vi "CountAndScan_v3.vi"() -> ()   [LabVIEW 2010]
uses:
  <vilib>/Utility/file.llb/Write To Spreadsheet File (DBL).vi
panel:
  out "Current-Calculated2":dbl caption="Current"
  out "Current-Calculated1":dbl caption="Current"
  in  "Timer":dbl=30.0 min=0.0 step=1.0
  out "Timer Progress":u8(slide)=29 scale=-1.1..4.0
  in  "SendMailAtEnd":bool=TRUE caption="at End"
  in  "SendMailAtEach":bool=TRUE caption="at Each Point"
  in  "SendMailAtStart":bool caption="at Start"
  out "Complete 2?":bool
  out "Homed ? 2":bool=TRUE caption="Homed ?"
  in  "MG17Motor 2":refnum<k7>(container)
  out "plStatusBits 2":i32=-1341913856
  out "Motor 2 error":errorcluster
  out "Motor 2":refnum<k7>
  out "plStatusBits":i32=-1341913856
  out "Homed ?":bool=TRUE
  out "Motor 1 error":errorcluster
  out "Motor 1":refnum<k7>
  in  "Beep":u16(ring)=1 items=["Off", "Each point", "End"]
  out "Aux":u64[](array[numeric])=[1279, 1631, 0]
  out "path":path=path "D:/Documents and Settings/All Users/Marcelo/Medidas/Paridade/2013-11-14 BBO/2013-11-13_97_placa_0.08gr_1200s.txt"
  out "Target 2":dbl caption="Target" format="%.2g"
  out "Current 2":sgl caption="APT-Current" format="%.2g"
  in  "Step 2":dbl caption="Step" min=0.3 max=360.0 step=1.0
  in  "Stop 2":dbl=50.0 caption="Stop" min=0.0 max=360.0 step=1.0
  in  "Start 2":dbl caption="Start" min=0.0 max=360.0 step=1.0
  out "Count 33":u32
  out "Count 32":u32
  out "Count 31":u32
  out "Count 23":u32
  out "Count 22":u32
  out "Count 21":u32
  out "Count 13":u32
  out "Count 12":u32=1631
  out "Count 11":u32=1279
  in  "stop":bool
  out "Target":dbl=19.0 format="%.2g"
  out "Complete 1?":bool=TRUE
  out "# of steps":dbl
  out "Current":sgl=18.999899 caption="APT-Current" format="%.2g"
  in  "Step":dbl=0.07999999821186066 min=0.02 max=360.0 step=1.0
  in  "Stop":dbl=19.08 min=0.0 max=360.0 step=1.0
  in  "Start":dbl=19.0 min=0.0 max=360.0 step=1.0
  in  "Serial Motor 2":i32=83829605 min=0 step=1
  in  "Serial Motor 1":i32=83830377 min=0 step=1
  in  "MG17Motor":refnum<k7>(container)
  out "ByteSize":u8=4
  in  "Sampling time":dbl=1200.0 min=0.0 step=1.0
  out "Handle 3":u32
  out "size(s)":i32=3
  out "Waveform Chart 9":u32(graph)
  out "Waveform Chart 8":u32(graph)
  out "Waveform Chart 7":u32(graph)
  out "Waveform Chart 6":u32(graph)
  out "Waveform Chart 5":u32(graph)
  out "Waveform Chart 4":u32(graph)
  out "Waveform Chart 3":u32(graph)
  out "Waveform Chart 2":u32(graph)=1631
  out "Waveform Chart 1":u32(graph)=1279
  in  "Plot 9":string(combo)="14"
  in  "Plot 8":string(combo)="8"
  in  "Plot 7":string(combo)="7"
  in  "Plot 6":string(combo)="6"
  in  "Plot 5":string(combo)="4"
  in  "Plot 4":string(combo)="3"
  in  "Plot 3":string(combo)="2"
  in  "Plot 2":string(combo)="1"
  in  "Plot 1":string(combo)="0"
  out "Delcom Serial Number":u32=20844 caption="20861"
  out "Handle":u32=17176
  out "2D Scan":bool
  out "Scan 2":bool
  out "Scan 1":bool=TRUE
  in  "Slide":dbl(slide)=1.0 min=0.0 max=2.0 step=1.0 scale=0.0..2.0
  in  "APD 4":bool
  in  "APD 3":bool
  in  "APD 2":bool=TRUE
  in  "APD 1":bool=TRUE
  # "FPGA SERIAL NUMBER"
  # "MOTOR 1"
  # "MOTOR 2"
  # "Send email"
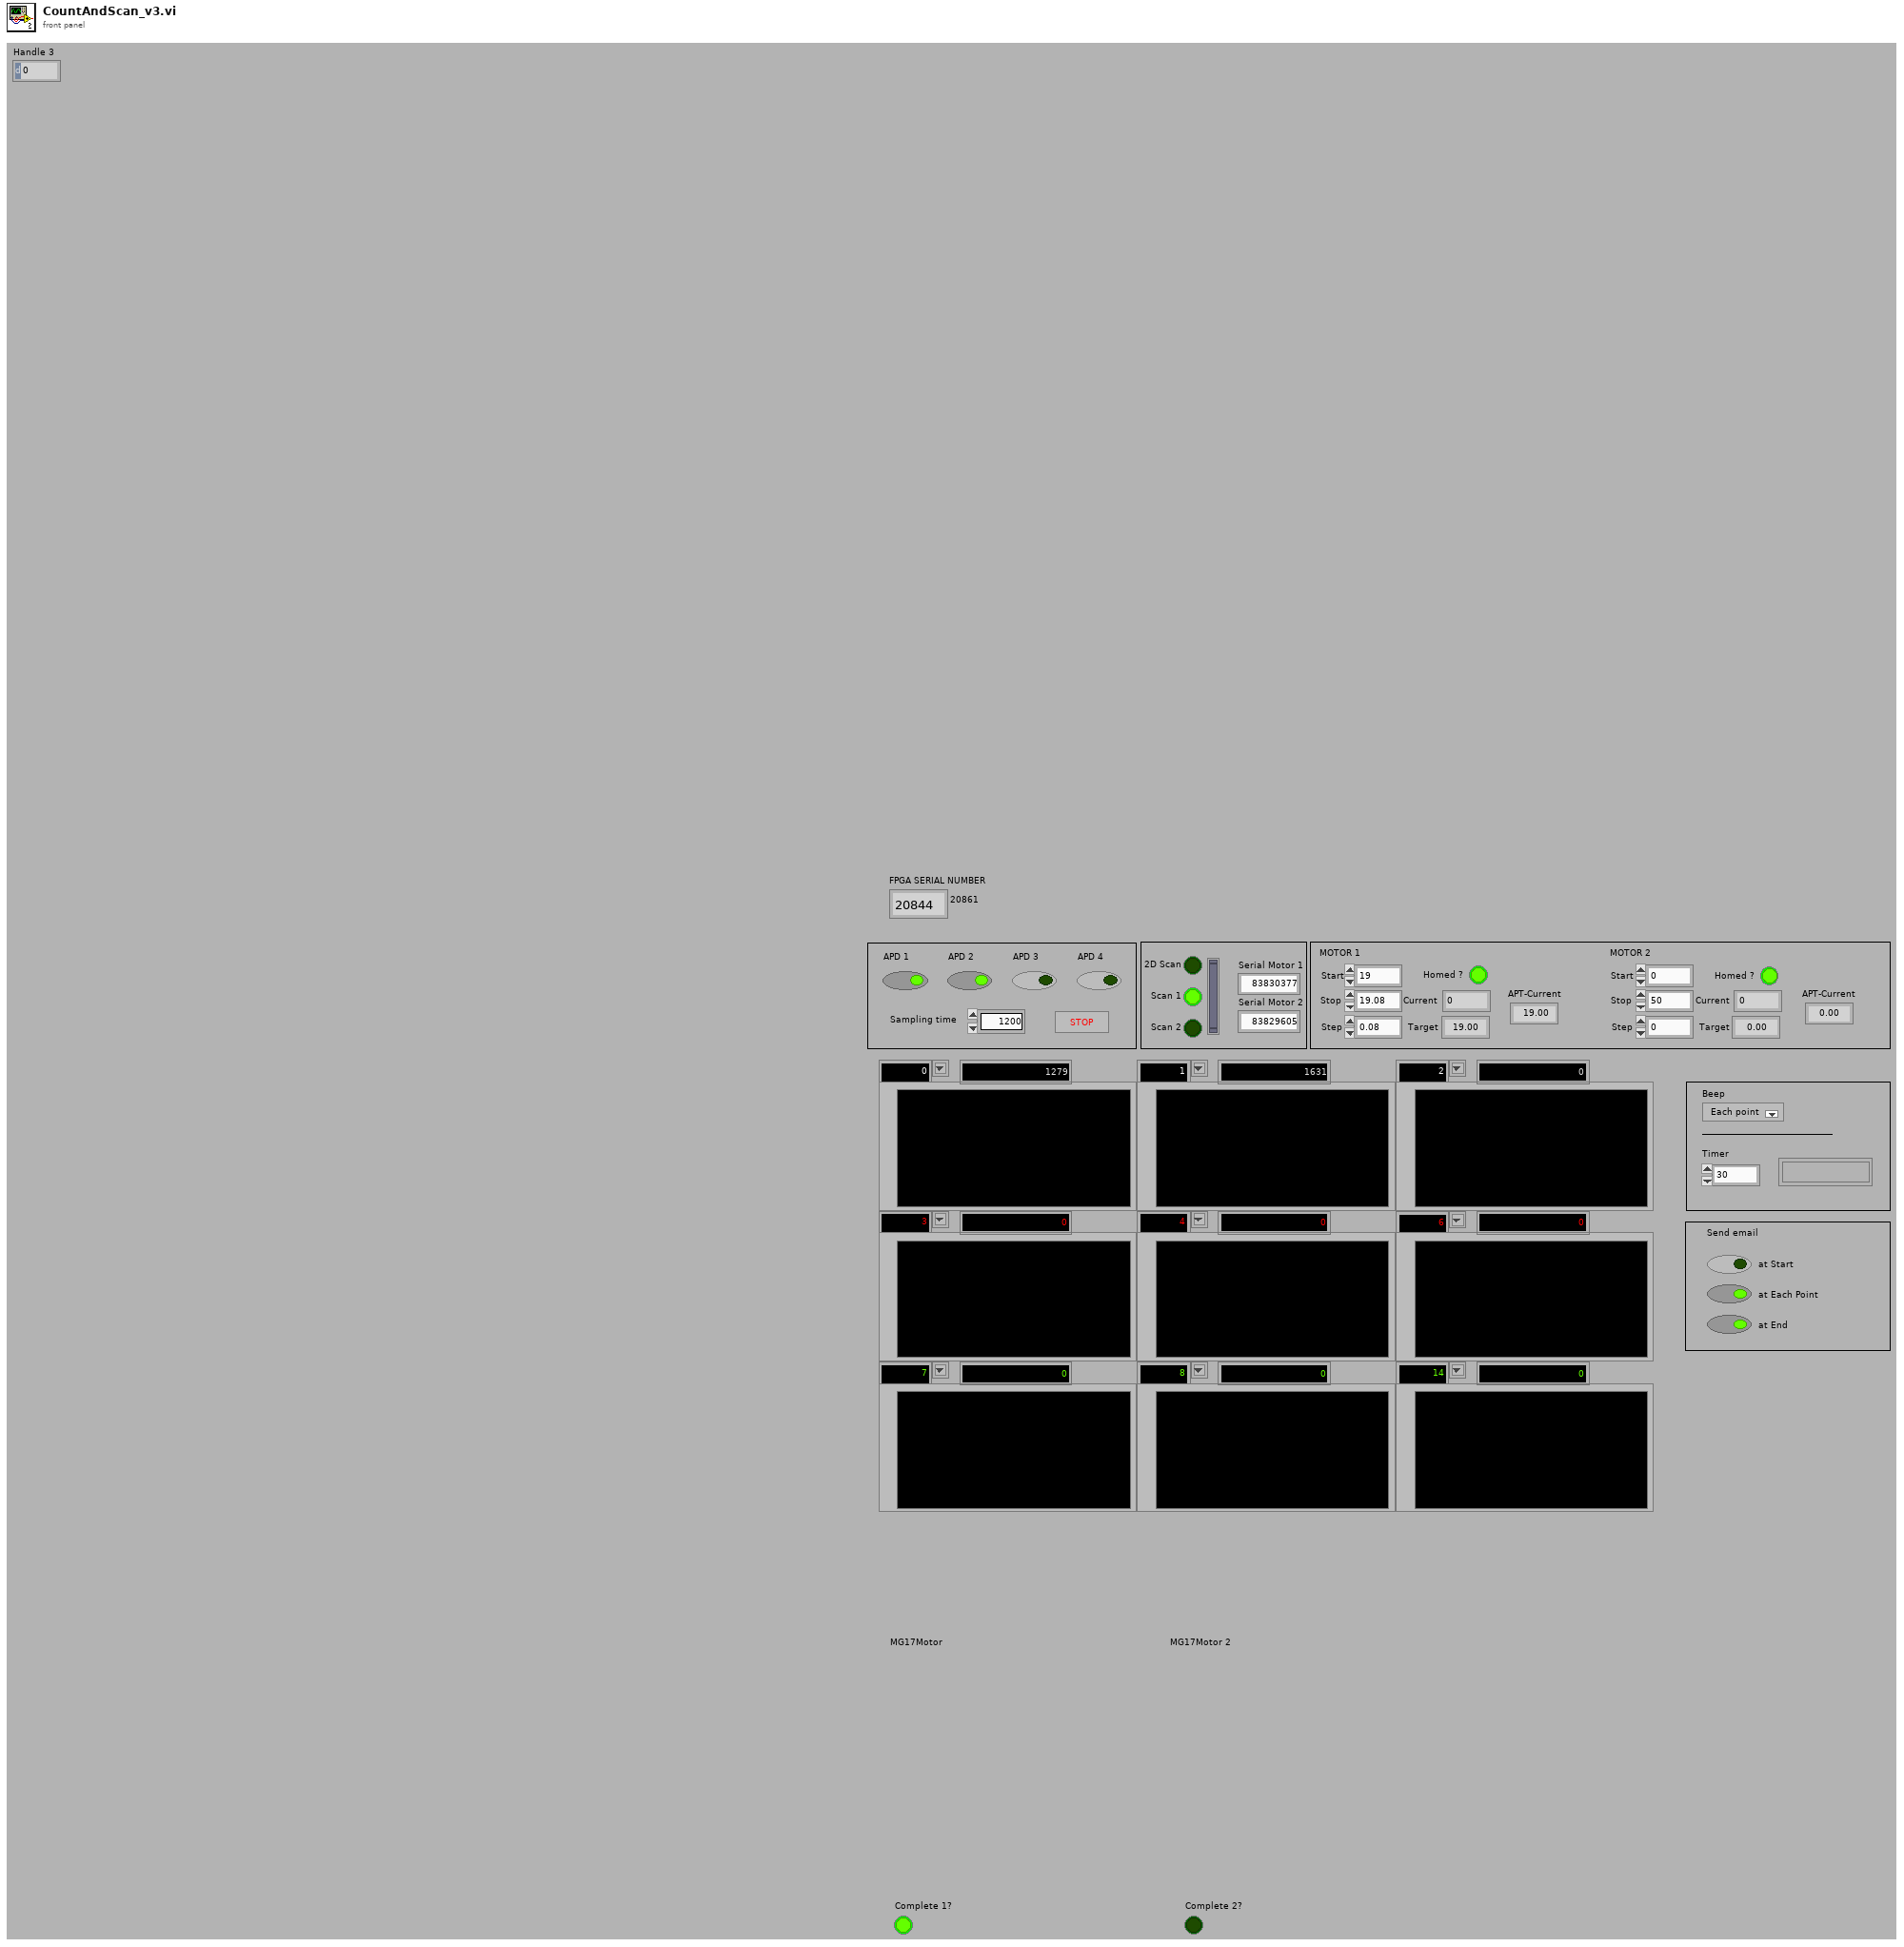
[diagram p1: front panel]
types:
  T1 = enum8{"Enabled", "Disabled", "Disabled and Grayed Out"}
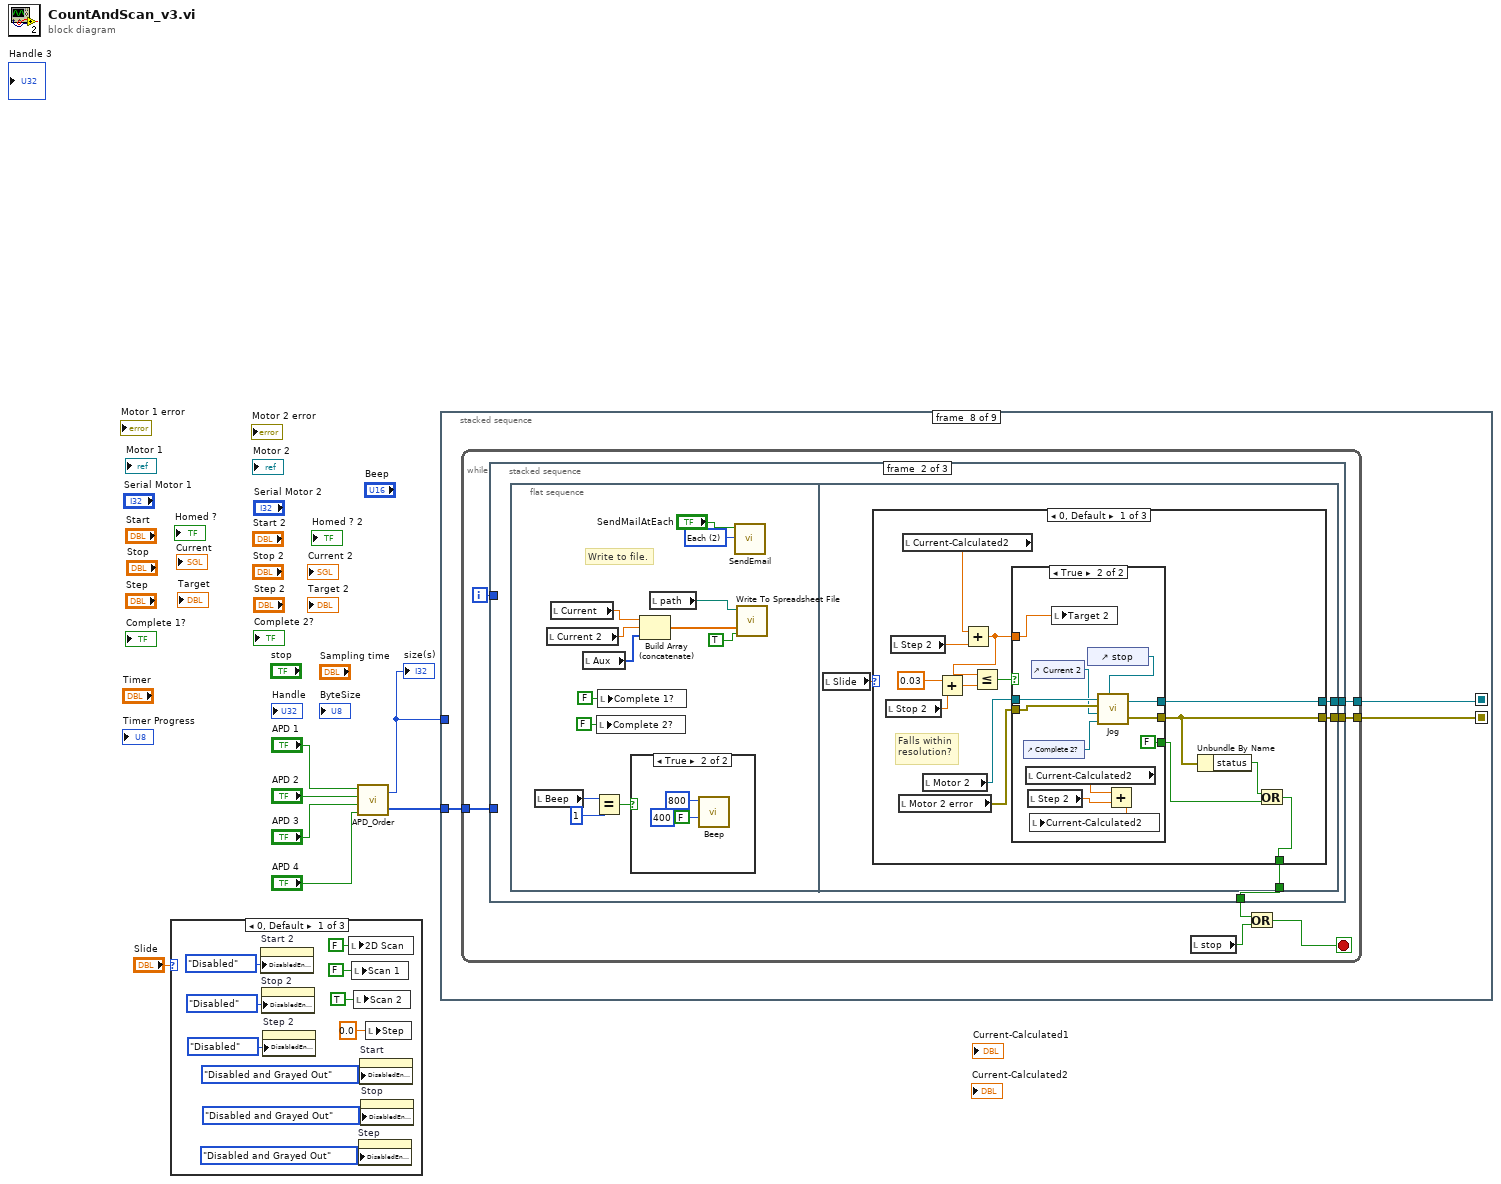
[diagram p0: block diagram]
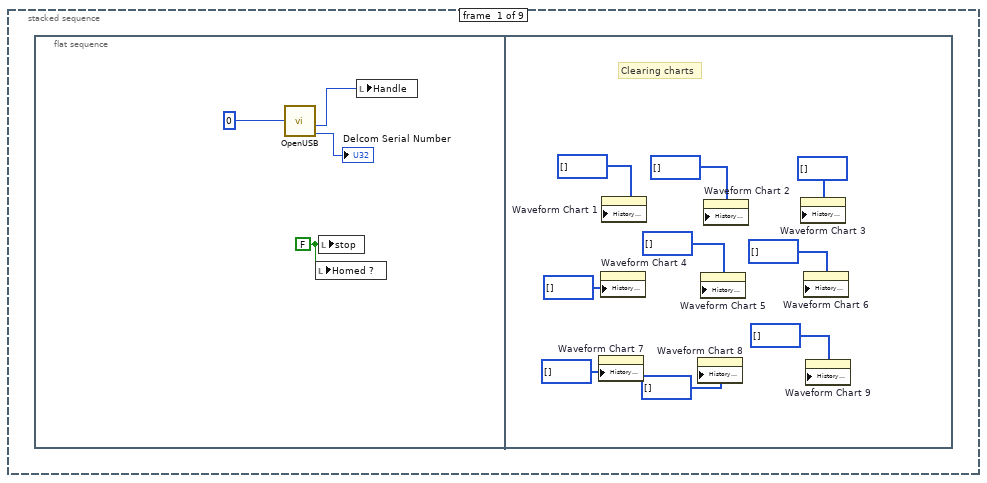
[diagram p2: hidden frame]
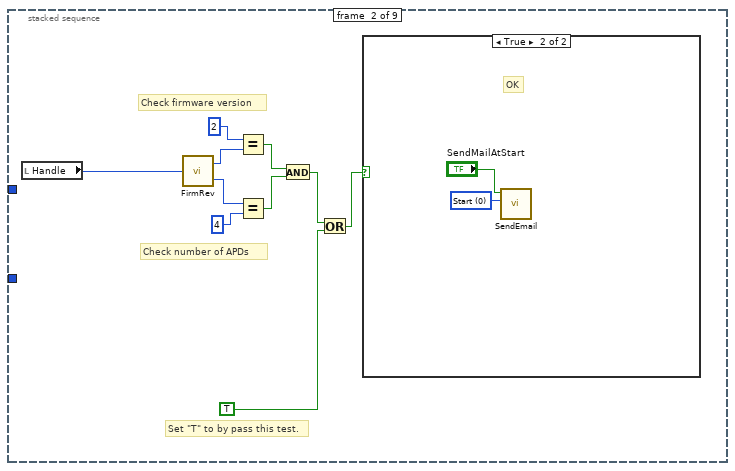
[diagram p3: hidden frame]
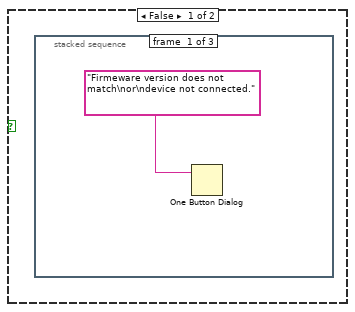
[diagram p4: hidden frame]
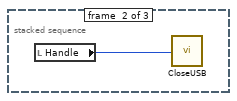
[diagram p5: hidden frame]
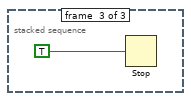
[diagram p6: hidden frame]
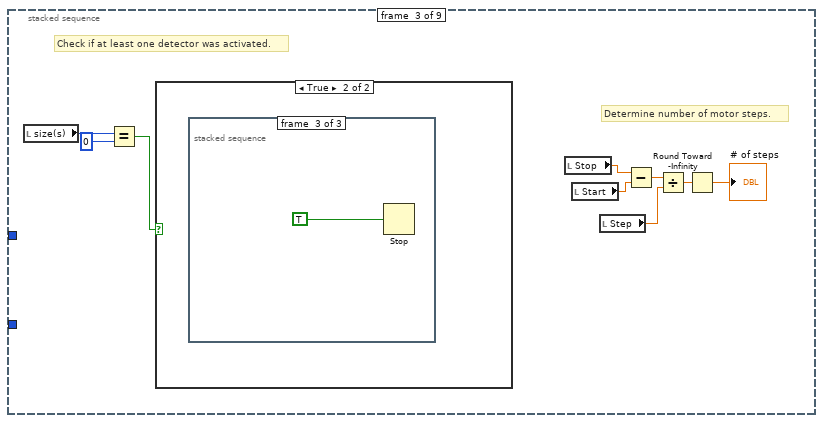
[diagram p7: hidden frame]
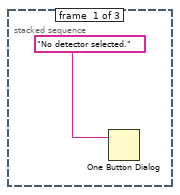
[diagram p9: hidden frame]
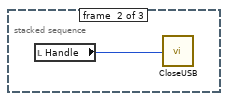
[diagram p10: hidden frame]
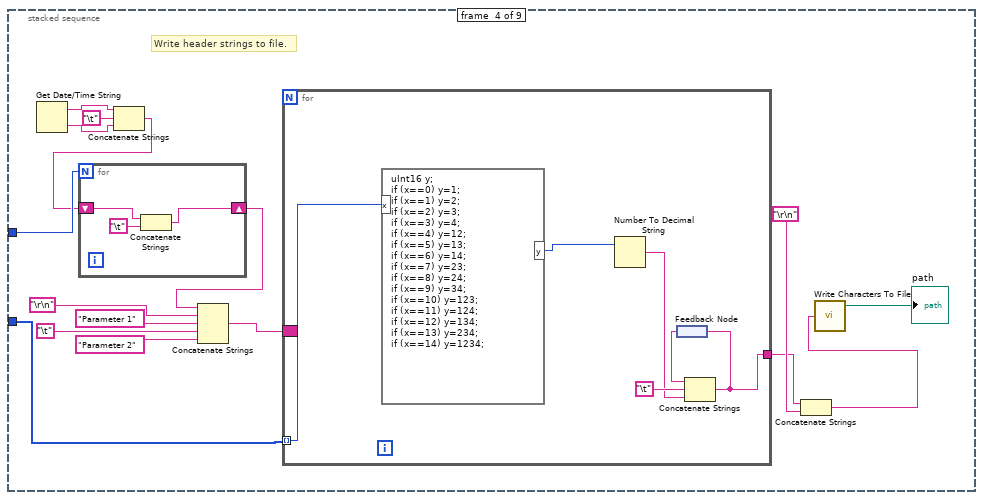
[diagram p11: hidden frame]
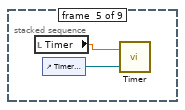
[diagram p12: hidden frame]
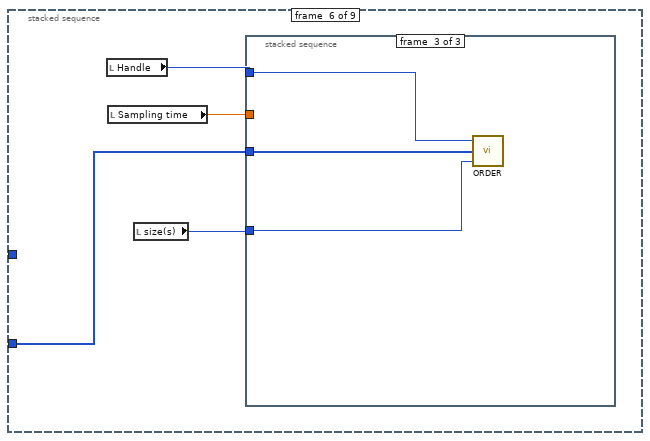
[diagram p13: hidden frame]
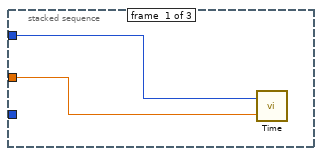
[diagram p14: hidden frame]
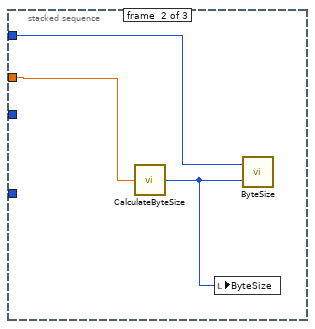
[diagram p15: hidden frame]
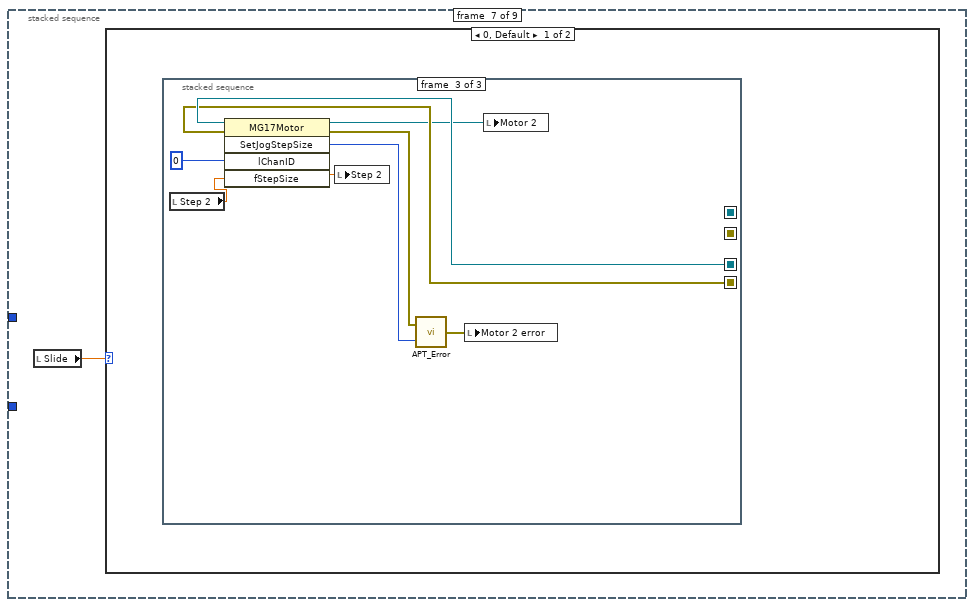
[diagram p16: hidden frame]
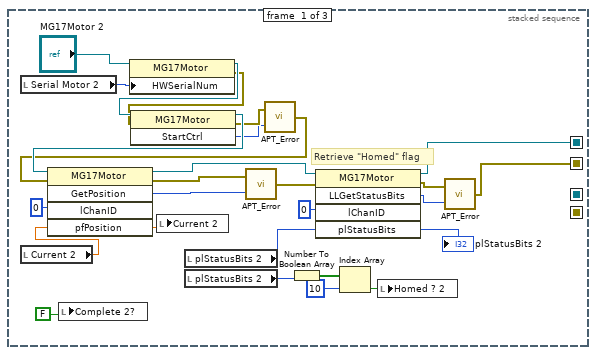
[diagram p17: hidden frame]
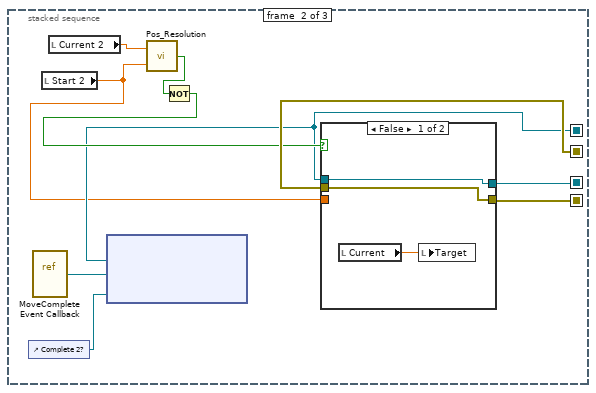
[diagram p18: hidden frame]
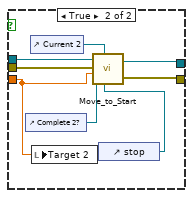
[diagram p19: hidden frame]
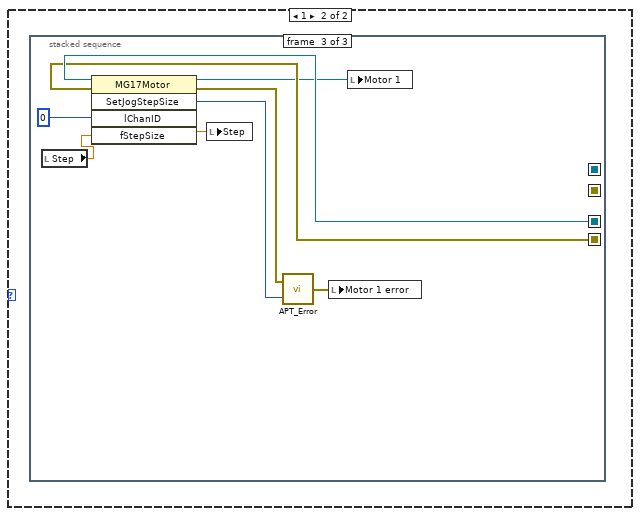
[diagram p20: hidden frame]
diagram:
  n1 = case shown="0, Default" "Slide" {
    frame 0, Default {
      n2 = property on="Start 2" class="DigNum (strict)"("DisabledEnum"=T1."Disabled" ("Disabled")) -> ()  [unwired: 2 in, 2 out]
      n3 = property on="Stop 2" class="DigNum (strict)"("DisabledEnum"=T1."Disabled" ("Disabled")) -> ()  [unwired: 2 in, 2 out]
      n4 = property on="Step 2" class="DigNum (strict)"("DisabledEnum"=T1."Disabled" ("Disabled")) -> ()  [unwired: 2 in, 2 out]
      n5 = local write "2D Scan"(FALSE ("Manual")) -> ()
      n6 = local write "Scan 1"(FALSE ("Scan 1")) -> ()
      n7 = local write "Scan 2"(TRUE ("Scan 2")) -> ()
      n8 = property on="Step" class="DigNum (strict)"("DisabledEnum"=T1."Disabled and Grayed Out" ("Disabled")) -> ()  [unwired: 2 in, 2 out]
      n9 = property on="Start" class="DigNum (strict)"("DisabledEnum"=T1."Disabled and Grayed Out" ("Disabled")) -> ()  [unwired: 2 in, 2 out]
      n10 = property on="Stop" class="DigNum (strict)"("DisabledEnum"=T1."Disabled and Grayed Out" ("Disabled")) -> ()  [unwired: 2 in, 2 out]
      n11 = local write "Step"(0.0 ("Step")) -> ()
    }
    frame 1 {
      n12 = property on="Start" class="DigNum (strict)"("DisabledEnum"=T1."Disabled" ("Disabled")) -> ()  [unwired: 2 in, 2 out]
      n13 = property on="Stop" class="DigNum (strict)"("DisabledEnum"=T1."Disabled" ("Disabled")) -> ()  [unwired: 2 in, 2 out]
      n14 = property on="Step" class="DigNum (strict)"("DisabledEnum"=T1."Disabled" ("Disabled")) -> ()  [unwired: 2 in, 2 out]
      n15 = property on="Start 2" class="DigNum (strict)"("DisabledEnum"=T1."Disabled and Grayed Out" ("Disabled")) -> ()  [unwired: 2 in, 2 out]
      n16 = property on="Stop 2" class="DigNum (strict)"("DisabledEnum"=T1."Disabled and Grayed Out" ("Disabled")) -> ()  [unwired: 2 in, 2 out]
      n17 = property on="Step 2" class="DigNum (strict)"("DisabledEnum"=T1."Disabled and Grayed Out" ("Disabled")) -> ()  [unwired: 2 in, 2 out]
      n18 = local write "Step 2"(0.0 ("Step 2")) -> ()
      n19 = local write "Scan 2"(FALSE ("Scan 2")) -> ()
      n20 = local write "2D Scan"(FALSE ("Manual")) -> ()
      n21 = local write "Scan 1"(TRUE ("Scan 1")) -> ()
    }
    frame 2 {
      "Scan 1" <- FALSE ("Scan 1")
      "2D Scan" <- TRUE ("Manual")
      "Scan 2" <- FALSE ("Scan 2")
    }
  }
  n22 = call "APD_Order.vi"("APD 4"="APD 4", "APD 3"="APD 3", "APD 2"="APD 2", "APD 1"="APD 1") -> ("Detectors"=w1:i32[], "size(s)"=w2:i32)
  "size(s)" <- w2
  n23 = stacked-sequence {
    seq-local: [_ _ _ _ _ _ _ w226 _] -> [_ _ _ _ _ _ _ _ w354]
    seq-local: [_ _ _ _ _ _ _ w225 _] -> [_ _ _ _ _ _ _ _ w353]
    tunnel: w2 -> [_ _ _ w80 _ _ _ _ _]
    tunnel: w1 -> [_ _ _ w73 _ w99 _ w227 _]
    frame #0 {
      n24 = flat-sequence {
        frame #0 {
          w31 = FALSE ("stop")
          n25 = call "OpenUSB.vi"("Device Number"=u32 0) -> ("Handle"=w32:u32, "Delcom Serial Number"=→"Delcom Serial Number":u32)  [unwired: 2 out]
          n26 = local write "Homed ?"(w31) -> ()
          n27 = local write "stop"(w31) -> ()
          n28 = local write "Handle"(w32) -> ()
        }
        frame #1 {
          # "Clearing charts"
          n29 = property on="Waveform Chart 7" class="WFChart (strict)"("History Data"=i32[] []) -> ()  [unwired: 2 in, 2 out]
          n30 = property on="Waveform Chart 4" class="WFChart (strict)"("History Data"=i32[] []) -> ()  [unwired: 2 in, 2 out]
          n31 = property on="Waveform Chart 1" class="WFChart (strict)"("History Data"=i32[] []) -> ()  [unwired: 2 in, 2 out]
          n32 = property on="Waveform Chart 8" class="WFChart (strict)"("History Data"=i32[] []) -> ()  [unwired: 2 in, 2 out]
          n33 = property on="Waveform Chart 5" class="WFChart (strict)"("History Data"=i32[] []) -> ()  [unwired: 2 in, 2 out]
          n34 = property on="Waveform Chart 2" class="WFChart (strict)"("History Data"=i32[] []) -> ()  [unwired: 2 in, 2 out]
          n35 = property on="Waveform Chart 3" class="WFChart (strict)"("History Data"=i32[] []) -> ()  [unwired: 2 in, 2 out]
          n36 = property on="Waveform Chart 6" class="WFChart (strict)"("History Data"=i32[] []) -> ()  [unwired: 2 in, 2 out]
          n37 = property on="Waveform Chart 9" class="WFChart (strict)"("History Data"=i32[] []) -> ()  [unwired: 2 in, 2 out]
        }
      }
    }
    frame #1 {
      # "Set \"T\" to by pass this test."
      # "Check number of APDs"
      # "Check firmware version"
      n38 = local read "Handle"() -> (w44:u32)
      n39 = call "FirmRev.vi"("Handle"=w44) -> ("Firmeware Version"=w45:u8, "APD nunmber"=w46:u8)
      n40 = Equal?(x=u8 2, y=w45) -> (x = y?=w49:bool)
      n41 = Equal?(x=w46, y=u8 4) -> (x = y?=w50:bool)
      n42 = And(x=w49, y=w50) -> (x .and. y?=w51:bool)
      n43 = Or(x=w51, y=TRUE) -> (x .or. y?=w52:bool)
      n44 = case shown="True" w52 {
        frame False {
          n45 = stacked-sequence {
            frame #0 {
              n46 = One Button Dialog(message="Firmeware version does not match\nor\ndevice not connected.") -> ()  [unwired: 1 in, 1 out]
            }
            frame #1 {
              n47 = local read "Handle"() -> (w55:u32)
              n48 = call "CloseUSB.vi"("Handle"=w55) -> ()  [unwired: 1 out]
            }
            frame #2 {
              n49 = Stop(stop? (T)=TRUE) -> ()
            }
          }
        }
        frame True {
          w58 = u16 0 items=["Start", "Stop", "Each"] ("Ring")
          # "OK"
          n50 = call "SendEmail.vi"("Send?"="SendMailAtStart", "Ring"=w58) -> ()  [unwired: 5 in]
        }
      }
    }
    frame #2 {
      # "Determine number of motor steps."
      # "Check if at least one detector was activated."
      n51 = local read "size(s)"() -> (w67:i32)
      n52 = Equal?(x=w67, y=0) -> (x = y?=w65:bool)
      n53 = case shown="True" w65 {
        frame False {
          # "PASS"
        }
        frame True {
          n54 = stacked-sequence {
            frame #0 {
              n55 = One Button Dialog(message="No detector selected.") -> ()  [unwired: 1 in, 1 out]
            }
            frame #1 {
              n56 = local read "Handle"() -> (w69:u32)
              n57 = call "CloseUSB.vi"("Handle"=w69) -> ()  [unwired: 1 out]
            }
            frame #2 {
              n58 = Stop(stop? (T)=TRUE) -> ()
            }
          }
        }
      }
      n59 = local read "Stop"() -> (w59:dbl)
      n60 = local read "Start"() -> (w64:dbl)
      n61 = local read "Step"() -> (w62:dbl)
      n62 = Subtract(x=w59, y=w64) -> (x-y=w63:dbl)
      n63 = Divide(x=w63, y=w62) -> (x/y=w61:dbl)
      n64 = Round Toward -Infinity(1:w61) -> (0:→"# of steps":dbl)
    }
    frame #3 {
      # "Write header strings to file."
      n65 = Get Date/Time String() -> (date string=w81:string, time string=w82:string)  [unwired: 3 in]
      n66 = Concatenate Strings(w81, "\t", w82) -> (w79:string)
      n67 = for {
        N: w80 -> [_]
        shift-right: [w94] -> w77
        shift-left: w79 -> [w93]
        n68 = Concatenate Strings(w93, "\t") -> (w94:string)
      }
      n69 = Concatenate Strings(w77, "\r\n", "Parameter 1", "\t", "Parameter 2") -> (w72:string)
      n70 = for {
        tunnel: [w91] -> w75
        border: w72 -> [_]
        tunnel: w73 -> [w87] mode=indexing
        n71 = formula code="uInt16 y;\nif (x==0) y=1;\nif (x==1) y=2;\nif (x==2) y=3;\nif (x==3) y=4;\nif (x==4) y=12;\nif (x==5) y=13;\nif (x==6) y=14;\nif (x==7) y=23;\nif (x==8) y=24;\nif (x==9) y=34;\nif (x==10) y=123;\nif (x==11) y=124;\nif (x==12) y=134;\nif (x==13) y=234;\nif (x==14) y=1234;"("x"=w87) -> ("y"=w89:u16)
        n72 = Number To Decimal String(number=w89) -> (decimal integer string=w88:string)  [unwired: 1 in]
        n73 = feedback #1() -> (w92:string)
        n74 = Concatenate Strings(w92, "\t", w88) -> (w91:string)
        n75 = feedback-in #1(w91) -> ()
      }
      n76 = Concatenate Strings(w75, "\r\n") -> (w74:string)
      n77 = call <vilib>:"Write Characters To File.vi"("character string"=w74) -> ("new file path (Not A Path if cancelled)"=→"path":path)  [unwired: 4 in]
    }
    frame #4 {
      n78 = local read "Timer"() -> (w96:dbl)
      n79 = control-ref of="Timer Progress"() -> (w97:refnum<vi>)
      n80 = call "Timer.vi"("Timer Progress"=w97, "Timer"=w96) -> ()  [unwired: 1 in]
    }
    frame #5 {
      n81 = local read "Handle"() -> (w101:u32)
      n82 = local read "Sampling time"() -> (w98:dbl)
      n83 = local read "size(s)"() -> (w100:i32)
      n84 = stacked-sequence {
        tunnel: w101 -> [w103 w106 w109]
        tunnel: w100 -> [_ _ w108]
        tunnel: w98 -> [w102 w105 _]
        tunnel: w99 -> [_ _ w107]
        frame #0 {
          n85 = call "Time.vi"("Time (s)"=w102, "Handle"=w103) -> ()  [unwired: 1 in]
        }
        frame #1 {
          n86 = call "CalculateByteSize.vi"("Tempo (s)"=w105) -> ("ByteSize"=w104:u8)
          n87 = local write "ByteSize"(w104) -> ()
          n88 = call "ByteSize.vi"("CounterByteSize"=w104, "Handle"=w106) -> ()  [unwired: 1 in]
        }
        frame #2 {
          n89 = call "ORDER.vi"("N"=w108, "Counter order"=w107, "Handle"=w109) -> ()  [unwired: 1 in]
        }
      }
    }
    frame #6 {
      n90 = local read "Slide"() -> (w110:dbl)
      n91 = case shown="0, Default" w110 {
        frame 0, Default {
          n92 = stacked-sequence {
            seq-local: [w119 _ _] -> [_ w141 _]
            seq-local: [w118 _ _] -> [_ w146 _]
            seq-local: [_ w143 _] -> [_ _ w167]
            seq-local: [_ w142 _] -> [_ _ w166]
            frame #0 {
              # "Retrieve \"Homed\" flag"
              n93 = local read "Serial Motor 2"() -> (w125:i32)
              n94 = local read "Current 2"() -> (w132:sgl)
              n95 = local write "Complete 2?"(FALSE ("Complete 1?")) -> ()
              n96 = property class="MG17Motor"(reference="MG17Motor 2", "HWSerialNum"=w125) -> (reference out=w136:refnum<k7>, error out=w135:errorcluster)  [unwired: 1 in]
              n97 = invoke class="MG17Motor" method="StartCtrl"(reference=w136, error in=w135) -> (reference out=w134:refnum<k7>, error out=w131:errorcluster, "StartCtrl"=w130:i32)  [unwired: 1 in]
              n98 = local read "plStatusBits 2"() -> (w113:i32)
              n99 = local read "plStatusBits 2"() -> (w111:i32)
              n100 = call "APT_Error.vi"("Return Code"=w130, "error in (no error)"=w131) -> ("error out"=w129:errorcluster)
              n101 = invoke class="MG17Motor" method="GetPosition"(reference=w134, error in=w129, "lChanID"=0, "pfPosition"=w132) -> (reference out=w123:refnum<k7>, error out=w128:errorcluster, "GetPosition"=w127:i32, "pfPosition"=w126:sgl)  [unwired: 1 in, 1 out]
              n102 = local write "Current 2"(w126) -> ()
              n103 = call "APT_Error.vi"("Return Code"=w127, "error in (no error)"=w128) -> ("error out"=w122:errorcluster)
              n104 = Number To Boolean Array(number=w111) -> (Boolean array=w116:bool[])
              n105 = invoke class="MG17Motor" method="LLGetStatusBits"(reference=w123, error in=w122, "lChanID"=0, "plStatusBits"=w113) -> (reference out=w119:refnum<k7>, error out=w120:errorcluster, "LLGetStatusBits"=w121:i32, "plStatusBits"=→"plStatusBits 2":i32)  [unwired: 1 in, 1 out]
              n106 = Index Array(array=w116, index=10) -> (element=w112:bool)
              n107 = local write "Homed ? 2"(w112) -> ()
              n108 = call "APT_Error.vi"("Return Code"=w121, "error in (no error)"=w120) -> ("error out"=w118:errorcluster)
            }
            frame #1 {
              n109 = control-ref of="Complete 2?"() -> (w140:refnum<vi>)
              n110 = vi-ref "MoveComplete Event Callback.vi"() -> ("vi reference"=w139:refnum<vi>)
              n111 = local read "Start 2"() -> (w138:dbl)
              n112 = local read "Current 2"() -> (w147:sgl)
              n113 = node(w141, w139, w140) -> ()  [unwired: 2 in, 2 out]
              n114 = call "Pos_Resolution.vi"("Target"=w138, "Current"=w147) -> ("Within resolution?"=w145:bool)
              n115 = Not(x=w145) -> (.not. x?=w144:bool)
              n116 = case shown="False" w144 {
                tunnel: w141 -> [w150 w157]
                tunnel: w146 -> [w149 w158]
                tunnel: [w150 w155] -> w143
                tunnel: [w149 w154] -> w142
                tunnel: w138 -> [_ w152]
                frame False {
                  n117 = local read "Current"() -> (w148:sgl)
                  n118 = local write "Target"(w148) -> ()
                }
                frame True {
                  n119 = control-ref of="Complete 2?"() -> (w153:refnum<vi>)
                  n120 = control-ref of="Current 2"() -> (w156:refnum<vi>)
                  n121 = local write "Target 2"(w152) -> ()
                  n122 = control-ref of="stop"() -> (w151:refnum<vi>)
                  n123 = call "Move_to_Start.vi"("Stop"=w151, "Current Pos"=w156, "Complete?"=w153, "Move To"=w152, "error in (no error)"=w158, "MG17Motor"=w157) -> ("error out"=w154:errorcluster, "reference out"=w155:refnum<k7>)
                }
              }
            }
            frame #2 {
              n124 = local read "Step 2"() -> (w163:dbl)
              n125 = invoke class="MG17Motor" method="SetJogStepSize"(reference=w167, error in=w166, "lChanID"=0, "fStepSize"=w163) -> (reference out=w162:refnum<k7>, error out=w161:errorcluster, "SetJogStepSize"=w160:i32, "fStepSize"=w164:sgl)  [unwired: 1 in, 1 out]
              n126 = local write "Step 2"(w164) -> ()
              n127 = call "APT_Error.vi"("Return Code"=w160, "error in (no error)"=w161) -> ("error out"=w159:errorcluster)
              n128 = local write "Motor 2 error"(w159) -> ()
              n129 = local write "Motor 2"(w162) -> ()
            }
          }
        }
        frame 1 {
          n130 = stacked-sequence {
            seq-local: [w176 _ _] -> [_ w198 _]
            seq-local: [w175 _ _] -> [_ w203 _]
            seq-local: [_ w200 _] -> [_ _ w224]
            seq-local: [_ w199 _] -> [_ _ w223]
            frame #0 {
              # "Retrieve \"Homed\" flag"
              n131 = local read "Serial Motor 1"() -> (w182:i32)
              n132 = local read "Current"() -> (w189:sgl)
              n133 = local write "Complete 1?"(FALSE ("Complete 1?")) -> ()
              n134 = property class="MG17Motor"(reference="MG17Motor", "HWSerialNum"=w182) -> (reference out=w193:refnum<k7>, error out=w192:errorcluster)  [unwired: 1 in]
              n135 = invoke class="MG17Motor" method="StartCtrl"(reference=w193, error in=w192) -> (reference out=w191:refnum<k7>, error out=w188:errorcluster, "StartCtrl"=w187:i32)  [unwired: 1 in]
              n136 = local read "plStatusBits"() -> (w170:i32)
              n137 = local read "plStatusBits"() -> (w168:i32)
              n138 = call "APT_Error.vi"("Return Code"=w187, "error in (no error)"=w188) -> ("error out"=w186:errorcluster)
              n139 = invoke class="MG17Motor" method="GetPosition"(reference=w191, error in=w186, "lChanID"=0, "pfPosition"=w189) -> (reference out=w180:refnum<k7>, error out=w185:errorcluster, "GetPosition"=w184:i32, "pfPosition"=w183:sgl)  [unwired: 1 in, 1 out]
              n140 = local write "Current"(w183) -> ()
              n141 = call "APT_Error.vi"("Return Code"=w184, "error in (no error)"=w185) -> ("error out"=w179:errorcluster)
              n142 = Number To Boolean Array(number=w168) -> (Boolean array=w173:bool[])
              n143 = invoke class="MG17Motor" method="LLGetStatusBits"(reference=w180, error in=w179, "lChanID"=0, "plStatusBits"=w170) -> (reference out=w176:refnum<k7>, error out=w177:errorcluster, "LLGetStatusBits"=w178:i32, "plStatusBits"=→"plStatusBits":i32)  [unwired: 1 in, 1 out]
              n144 = Index Array(array=w173, index=10) -> (element=w169:bool)
              n145 = local write "Homed ?"(w169) -> ()
              n146 = call "APT_Error.vi"("Return Code"=w178, "error in (no error)"=w177) -> ("error out"=w175:errorcluster)
            }
            frame #1 {
              n147 = control-ref of="Complete 1?"() -> (w197:refnum<vi>)
              n148 = vi-ref "MoveComplete Event Callback.vi"() -> ("vi reference"=w196:refnum<vi>)
              n149 = local read "Start"() -> (w195:dbl)
              n150 = local read "Current"() -> (w204:sgl)
              n151 = node(w198, w196, w197) -> ()  [unwired: 2 in, 2 out]
              n152 = call "Pos_Resolution.vi"("Target"=w195, "Current"=w204) -> ("Within resolution?"=w202:bool)
              n153 = Not(x=w202) -> (.not. x?=w201:bool)
              n154 = case shown="True" w201 {
                tunnel: w198 -> [w207 w214]
                tunnel: w203 -> [w206 w215]
                tunnel: [w207 w212] -> w200
                tunnel: [w206 w211] -> w199
                tunnel: w195 -> [_ w209]
                frame False {
                  n155 = local read "Current"() -> (w205:sgl)
                  n156 = local write "Target"(w205) -> ()
                }
                frame True {
                  n157 = control-ref of="Complete 1?"() -> (w210:refnum<vi>)
                  n158 = control-ref of="Current"() -> (w213:refnum<vi>)
                  n159 = local write "Target"(w209) -> ()
                  n160 = control-ref of="stop"() -> (w208:refnum<vi>)
                  n161 = call "Move_to_Start.vi"("Stop"=w208, "Current Pos"=w213, "Complete?"=w210, "Move To"=w209, "error in (no error)"=w215, "MG17Motor"=w214) -> ("error out"=w211:errorcluster, "reference out"=w212:refnum<k7>)
                }
              }
            }
            frame #2 {
              n162 = local read "Step"() -> (w220:dbl)
              n163 = invoke class="MG17Motor" method="SetJogStepSize"(reference=w224, error in=w223, "lChanID"=0, "fStepSize"=w220) -> (reference out=w219:refnum<k7>, error out=w218:errorcluster, "SetJogStepSize"=w217:i32, "fStepSize"=w221:sgl)  [unwired: 1 in, 1 out]
              n164 = local write "Step"(w221) -> ()
              n165 = call "APT_Error.vi"("Return Code"=w217, "error in (no error)"=w218) -> ("error out"=w216:errorcluster)
              n166 = local write "Motor 1 error"(w216) -> ()
              n167 = local write "Motor 1"(w219) -> ()
            }
          }
        }
      }
    }
    frame #7 {
      n168 = while {
        tunnel: w227 -> [w233]
        tunnel: [w229] -> w226
        tunnel: [w228] -> w225
        i -> [w234]
        stop <- w230 stop-if-true
        n169 = stacked-sequence {
          tunnel: w234 -> [w255 _ _]
          tunnel: w233 -> [w245 _ _]
          tunnel: [_ w262 _] -> w232
          tunnel: [_ w261 _] -> w229
          tunnel: [_ w260 _] -> w228
          frame #0 {
            # "Updates photon counts indicators."
            n170 = local read "Sampling time"() -> (w258:dbl)
            n171 = local read "ByteSize"() -> (w257:u8)
            n172 = local read "size(s)"() -> (w256:i32)
            n173 = local read "Handle"() -> (w259:u32)
            n174 = call "COUNTandREAD.vi"("i"=w255, "Byte size"=w257, "Num. of Counters"=w256, "tempo (s)"=w258, "handle"=w259) -> ("Output"=w235:u64[])  [unwired: 1 in]
            "Aux" <- w235
            n175 = call "Get_Element.vi"("Search for string"="Plot 7", "Det. list"=w245, "Meas. Data"=w235) -> ("Output"=→"Waveform Chart 7" →"Count 31":u32)
            n176 = call "Get_Element.vi"("Search for string"="Plot 4", "Det. list"=w245, "Meas. Data"=w235) -> ("Output"=→"Waveform Chart 4" →"Count 21":u32)
            n177 = call "Get_Element.vi"("Search for string"="Plot 1", "Det. list"=w245, "Meas. Data"=w235) -> ("Output"=→"Waveform Chart 1" →"Count 11":u32)
            n178 = call "Get_Element.vi"("Search for string"="Plot 8", "Det. list"=w245, "Meas. Data"=w235) -> ("Output"=→"Waveform Chart 8" →"Count 32":u32)
            n179 = call "Get_Element.vi"("Search for string"="Plot 2", "Det. list"=w245, "Meas. Data"=w235) -> ("Output"=→"Waveform Chart 2" →"Count 12":u32)
            n180 = call "Get_Element.vi"("Search for string"="Plot 5", "Det. list"=w245, "Meas. Data"=w235) -> ("Output"=→"Waveform Chart 5" →"Count 22":u32)
            n181 = call "Get_Element.vi"("Search for string"="Plot 9", "Det. list"=w245, "Meas. Data"=w235) -> ("Output"=→"Waveform Chart 9" →"Count 33":u32)
            n182 = call "Get_Element.vi"("Search for string"="Plot 6", "Det. list"=w245, "Meas. Data"=w235) -> ("Output"=→"Waveform Chart 6" →"Count 23":u32)
            n183 = call "Get_Element.vi"("Search for string"="Plot 3", "Det. list"=w245, "Meas. Data"=w235) -> ("Output"=→"Waveform Chart 3" →"Count 13":u32)
          }
          frame #1 {
            n184 = flat-sequence {
              tunnel: [w281] -> w262
              tunnel: [w280] -> w261
              tunnel: [w279] -> w260
              frame #0 {
                w263 = u16 2 items=["Start", "Stop", "Each"] ("Ring")
                # "Write to file."
                n185 = local read "Beep"() -> (w268:u16)
                n186 = local read "Current 2"() -> (w272:sgl)
                n187 = local read "Current"() -> (w273:sgl)
                n188 = local read "Aux"() -> (w271:u64[])
                n189 = Equal?(x=w268, y=u16 1) -> (x = y?=w266:bool)
                n190 = local write "Complete 2?"(FALSE ("Complete 1?")) -> ()
                n191 = local write "Complete 1?"(FALSE ("Complete 1?")) -> ()
                n192 = case shown="True" w266 {
                  frame False {
                  }
                  frame True {
                    n193 = call <vilib>:"Beep.vi"("use system alert? (T)"=FALSE, "duration (msec)"=u32 400, "frequency (Hz)"=u32 800) -> ()  [unwired: 9 in]
                  }
                }
                n194 = Build Array (concatenate)(w273, w272, w271) -> (w270:sgl[])
                n195 = local read "path"() -> (w275:path)
                n196 = call "SendEmail.vi"("Send?"="SendMailAtEach", "Ring"=w263) -> ()  [unwired: 5 in]
                n197 = call-poly <vilib>:"Write To Spreadsheet File.vi"("append to file? (new file:F)"=TRUE, "1D data"=w270, "file path (dialog if empty)"=w275) -> ()  [unwired: 5 in, 1 out]
              }
              frame #1 {
                n198 = local read "Slide"() -> (w282:dbl)
                n199 = case shown="0, Default" w282 {
                  tunnel: [w287 w316 FALSE ("status")] -> w281
                  tunnel: [w291 w320 refnum<k7> refnum ("reference out")] -> w280
                  tunnel: [w290 w319 errorcluster {"status"=FALSE, "code"=0, "source"=""} ("error out")] -> w279
                  frame 0, Default {
                    # "Falls within\nresolution?"
                    n200 = local read "Stop 2"() -> (w285:dbl)
                    n201 = local read "Step 2"() -> (w296:dbl)
                    n202 = local read "Motor 2 error"() -> (w292:errorcluster)
                    n203 = local read "Current-Calculated2"() -> (w283:dbl)
                    n204 = local read "Motor 2"() -> (w293:refnum<k7>)
                    n205 = Add(x=0.03, y=w285) -> (x+y=w284:dbl)
                    n206 = Add(x=w283, y=w296) -> (x+y=w294:dbl)
                    n207 = Less Or Equal?(x=w294, y=w284) -> (x <= y?=w295:bool)
                    n208 = case shown="True" w295 {
                      tunnel: w294 -> [_ w303]
                      tunnel: w293 -> [w298 w311]
                      tunnel: w292 -> [w297 w310]
                      tunnel: [w298 w306] -> w291
                      tunnel: [w297 w305] -> w290
                      tunnel: [TRUE FALSE] -> w289
                      frame False {
                      }
                      frame True {
                        n209 = control-ref of="Complete 2?"() -> (w308:refnum<vi>)
                        n210 = local read "Current-Calculated2"() -> (w302:dbl)
                        n211 = local read "Step 2"() -> (w301:dbl)
                        n212 = control-ref of="Current 2"() -> (w309:refnum<vi>)
                        n213 = local write "Target 2"(w303) -> ()
                        n214 = control-ref of="stop"() -> (w307:refnum<vi>)
                        n215 = call "Jog.vi"("MG17Motor"=w311, "error in (no error)"=w310, "Current Pos"=w309, "Complete?"=w308, "Stop"=w307) -> ("reference out"=w306:refnum<k7>, "error out"=w305:errorcluster)
                        n216 = Add(x=w302, y=w301) -> (x+y=w300:dbl)
                        n217 = local write "Current-Calculated2"(w300) -> ()
                      }
                    }
                    n218 = Unbundle By Name(w290) -> ("status"=w288:bool)
                    n219 = Or(x=w288, y=w289) -> (x .or. y?=w287:bool)
                  }
                  frame 1 {
                    # "Falls within\nresolution?"
                    n220 = local read "Current-Calculated1"() -> (w312:dbl)
                    n221 = local read "Stop"() -> (w314:dbl)
                    n222 = local read "Step"() -> (w325:dbl)
                    n223 = local read "Motor 1 error"() -> (w321:errorcluster)
                    n224 = local read "Motor 1"() -> (w322:refnum<k7>)
                    n225 = Add(x=0.03, y=w314) -> (x+y=w313:dbl)
                    n226 = Add(x=w312, y=w325) -> (x+y=w323:dbl)
                    n227 = Less Or Equal?(x=w323, y=w313) -> (x <= y?=w324:bool)
                    n228 = case shown="True" w324 {
                      tunnel: w323 -> [_ w332]
                      tunnel: w322 -> [w327 w340]
                      tunnel: w321 -> [w326 w339]
                      tunnel: [w327 w335] -> w320
                      tunnel: [w326 w334] -> w319
                      tunnel: [TRUE FALSE] -> w318
                      frame False {
                      }
                      frame True {
                        n229 = local read "Current-Calculated1"() -> (w331:dbl)
                        n230 = control-ref of="Complete 1?"() -> (w337:refnum<vi>)
                        n231 = local read "Step"() -> (w330:dbl)
                        n232 = control-ref of="Current"() -> (w338:refnum<vi>)
                        n233 = local write "Target"(w332) -> ()
                        n234 = control-ref of="stop"() -> (w336:refnum<vi>)
                        n235 = call "Jog.vi"("MG17Motor"=w340, "error in (no error)"=w339, "Current Pos"=w338, "Complete?"=w337, "Stop"=w336) -> ("reference out"=w335:refnum<k7>, "error out"=w334:errorcluster)
                        n236 = Add(x=w331, y=w330) -> (x+y=w329:dbl)
                        n237 = local write "Current-Calculated1"(w329) -> ()
                      }
                    }
                    n238 = Unbundle By Name(w319) -> ("status"=w317:bool)
                    n239 = Or(x=w317, y=w318) -> (x .or. y?=w316:bool)
                  }
                  frame 2 {
                    # "Temporary code. It is to be modified when\nraster scan is included."
                  }
                }
              }
            }
          }
          frame #2 {
            n240 = Wait (ms)(milliseconds to wait=u32 1000) -> ()  [unwired: 1 out]
          }
        }
        n241 = local read "stop"() -> (w231:bool)
        n242 = Or(x=w232, y=w231) -> (x .or. y?=w230:bool)
      }
    }
    frame #8 {
      w345 = u16 1 items=["Start", "Stop", "Each"] ("Ring")
      n243 = local read "Beep"() -> (w352:u16)
      n244 = local read "stop"() -> (w348:bool)
      n245 = Not(x=w348) -> (.not. x?=w347:bool)
      n246 = Equal?(x=w352, y=u16 2) -> (x = y?=w350:bool)
      n247 = property on="Start" class="DigNum (strict)"("DisabledEnum"=T1."Enabled" ("Disabled")) -> ()  [unwired: 2 in, 2 out]
      n248 = property on="Stop" class="DigNum (strict)"("DisabledEnum"=T1."Enabled" ("Disabled")) -> ()  [unwired: 2 in, 2 out]
      n249 = property on="Step" class="DigNum (strict)"("DisabledEnum"=T1."Enabled" ("Disabled")) -> ()  [unwired: 2 in, 2 out]
      n250 = And(x=w350, y=w347) -> (x .and. y?=w349:bool)
      n251 = case shown="True" w349 {
        frame False {
        }
        frame True {
          n252 = call <vilib>:"Beep.vi"("use system alert? (T)"=FALSE, "duration (msec)"=u32 400, "frequency (Hz)"=u32 800) -> ()  [unwired: 9 in]
        }
      }
      n253 = local read "Handle"() -> (w361:u32)
      n254 = property on="Start 2" class="DigNum (strict)"("DisabledEnum"=T1."Enabled" ("Disabled")) -> ()  [unwired: 2 in, 2 out]
      n255 = property on="Step 2" class="DigNum (strict)"("DisabledEnum"=T1."Enabled" ("Disabled")) -> ()  [unwired: 2 in, 2 out]
      n256 = property on="Stop 2" class="DigNum (strict)"("DisabledEnum"=T1."Enabled" ("Disabled")) -> ()  [unwired: 2 in, 2 out]
      n257 = call "CloseUSB.vi"("Handle"=w361) -> ()  [unwired: 1 out]
      n258 = call "SendEmail.vi"("Send?"="SendMailAtEnd", "Ring"=w345) -> ()  [unwired: 5 in]
      n259 = invoke class="MG17Motor" method="StopCtrl"(reference=w354, error in=w353) -> ()  [unwired: 1 in, 3 out]
    }
  }
